vi "Dialog Tester - Plain PopUp.vi"() -> ()   [LabVIEW 2021]
doc: "Test the plain/simple pop up types"
uses:
  Theme/Dialog colors--typedef.ctl
  Theme/Button colors--typedef.ctl
  Theme/Theme.lvclass/Theme.ctl
  Popup/PopUp Theme Global.vi
  Theme/Theme.lvclass
  Plain/Plain - One Button/Plain - One Button.lvclass
  Plain/Plain - Two Button/Plain - Two Button.lvclass
  Plain/Plain - Three Button/Plain - Three Button.lvclass
panel:
  in  "button colors":T1={"false color"={"border"=13816530, "fill"=14869218}, "hover color"={"border"=11908533, "fill"=16447999}, "press color"={"border"=0, "fill"=11908533}, "Boolean Text"=1668818, "Text.Font Name"="Segoe UI", "Text.Font Size"=20, "Bold?"=TRUE, "Itallic?"=FALSE}
  in  "keep transparent buttons?":bool=TRUE
  in  "dialog colors":T2={"Header"=1668818, "Background"=15790320, "Picture Background"=16777216}
  out "choice":u8
  out "Choice":bool
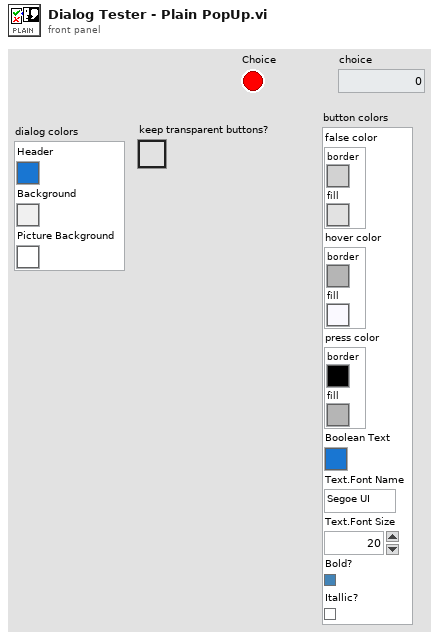
[diagram p1: front panel]
types:
  T1 = typedef "Theme.lvclass/Button colors--typedef.ctl" = cluster{"false color":cluster{"border":u32, "fill":u32}, "hover color":cluster{"border":u32, "fill":u32}, "press color":cluster{"border":u32, "fill":u32}, "Boolean Text":u32, "Text.Font Name":string, "Text.Font Size":u32, "Bold?":bool, "Itallic?":bool}
  T2 = typedef "Theme.lvclass/Dialog colors--typedef.ctl" = cluster{"Header":u32, "Background":u32, "Picture Background":u32}
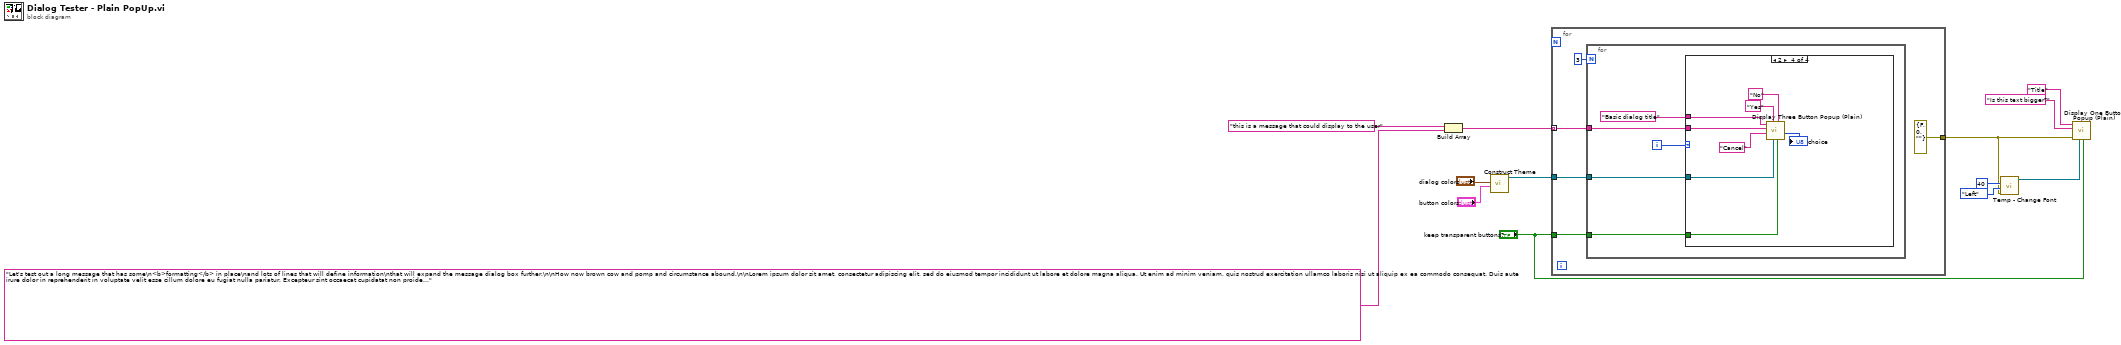
[diagram p0: block diagram]
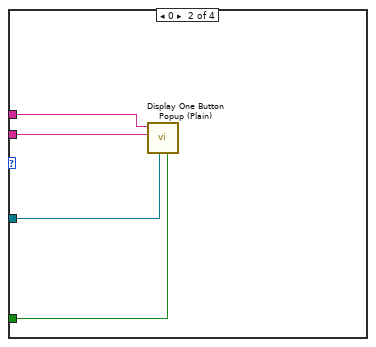
[diagram p3: hidden frame]
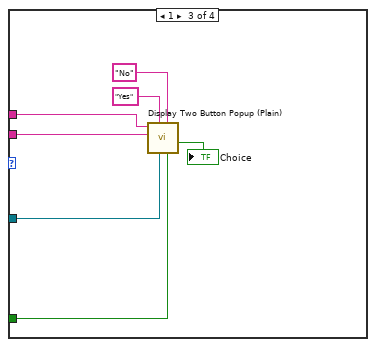
[diagram p4: hidden frame]
diagram:
  n1 = Build Array("this is a message that could display to the user" ("Message"), "Let's test out a long message that has some\n<b>formatting</b> in place\nand lots of lines that will define information\nthat will expand the message dialog box further.\n\nHow now brown cow and pomp and circumstance abound.\n\nLorem ipsum dolor sit amet, consectetur adipiscing elit, sed do eiusmod tempor incididunt ut labore et dolore magna aliqua. Ut enim ad minim veniam, quis nostrud exercitation ullamco laboris nisi ut aliquip ex ea commodo consequat. Duis aute irure dolor in reprehenderit in voluptate velit esse cillum dolore eu fugiat nulla pariatur. Excepteur sint occaecat cupidatat non proident, sunt in culpa qui officia deserunt mollit anim id est laborum." ("Message")) -> (w11:string[])
  n2 = call "Construct Theme.vi"("button colors"="button colors", "dialog colors"="dialog colors") -> ("Theme out"=w13:refnum<class "Theme.lvclass">)  [unwired: 8 in, 1 out]
  n3 = for {
    tunnel: w13 -> [w18]
    tunnel: w11 -> [w16] mode=indexing
    tunnel: [errorcluster {"status"=FALSE, "code"=0, "source"=""} ("error constant")] -> w4
    tunnel: "keep transparent buttons?" -> [w14]
    n4 = for {
      N: 3 -> [_]
      tunnel: w18 -> [w23]
      tunnel: w16 -> [w20]
      tunnel: w14 -> [w19]
      i -> [w21]
      n5 = case shown="2" w21 {
        tunnel: w23 -> [_ w27 w34 w42]
        tunnel: "Basic dialog title" ("Dialog Title") -> [_ w26 w33 w41]
        tunnel: w20 -> [_ w25 w32 w40]
        tunnel: w19 -> [_ w24 w28 w35]
        frame Default {
        }
        frame 0 {
          n6 = call "Display One Button Popup (Plain).vi"("keep transparent buttons?"=w24, "Theme"=w27, "Message"=w25, "Dialog Title"=w26) -> ()  [unwired: 7 in, 1 out]
        }
        frame 1 {
          n7 = call "Display Two Button Popup (Plain).vi"("keep transparent buttons?"=w28, "N-Text"="No", "Theme"=w34, "Y-Text"="Yes", "Message"=w32, "Dialog Title"=w33) -> ("Choice"=→"Choice":bool)  [unwired: 4 in, 1 out]
        }
        frame 2 {
          n8 = call "Display Three Button Popup (Plain).vi"("keep transparent buttons?"=w35, "Action 1 Text"="No" ("N-Text"), "Theme"=w42, "Action 0 Text"="Yes" ("Y-Text"), "Action 2 Text"="Cancel" ("Action 3 Text"), "Message"=w40, "Dialog Title"=w41) -> ("Choice"=→"choice":u8)  [unwired: 3 in, 1 out]
        }
      }
    }
  }
  n9 = call "Temp - Change Font.vi"("error in (no error)"=w4, "message font.Text.Justification"=enum16{"Left", "Center", "Right"}."Left", "message font.Text.Font Size"=u32 40) -> ("Theme out"=w6:refnum<class "Theme.lvclass">)  [unwired: 7 in, 1 out]
  n10 = call "Display One Button Popup (Plain).vi"("keep transparent buttons?"="keep transparent buttons?", "Theme"=w6, "error in"=w4, "Message"="Is this text bigger?", "Dialog Title"="Title") -> ()  [unwired: 6 in, 1 out]
